vi "Read Write Script 2.vi"(5 "# of Words":i32, 6 "chip select (0)":u32, 7 "Write register":u8, 8 "error in (no error)":errorcluster, 9 "Write Data":u8[][](array[numeric]), 10 "delay in milliseconds (0)":u8, 11 "spi script reference in":T1) -> (0 "error out":errorcluster, 1 "script read index":u32, 3 "spi script reference out":T1)   [LabVIEW 2013]
uses:
  <vilib>/ni845x/ni845x.llb/ni845xSpiScriptControl.ctl
  <vilib>/ni845x/ni845x.llb/NI-845x SPI Script Ms Delay.vi
panel:
  out "data set":u8[](array[numeric])
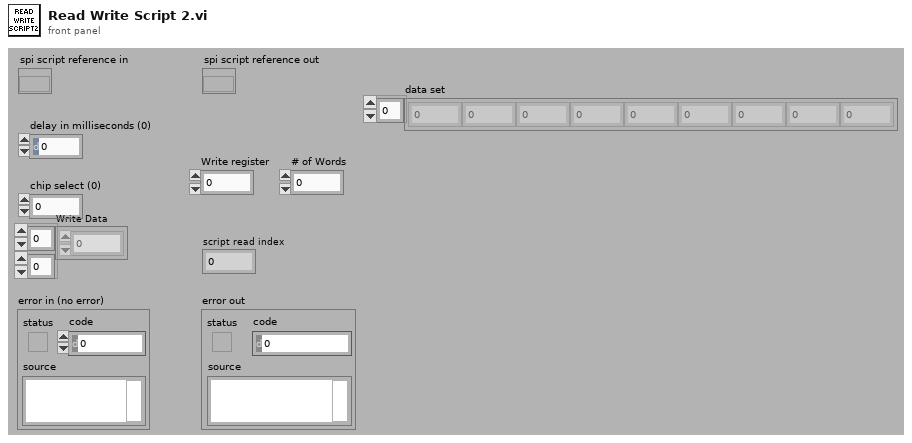
[diagram p1: front panel]
types:
  T1 = typedef "ni845xSpiScriptControl.ctl" = refnum<k20>
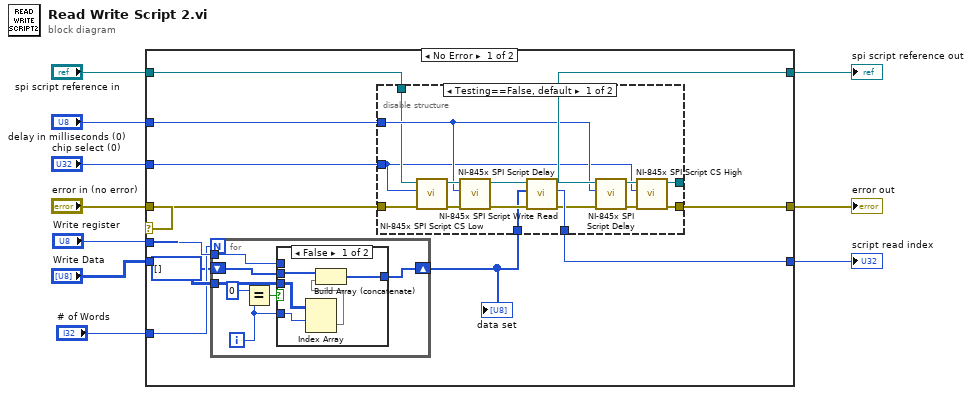
[diagram p0: block diagram]
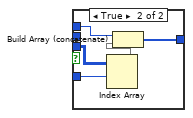
[diagram p2: hidden frame]
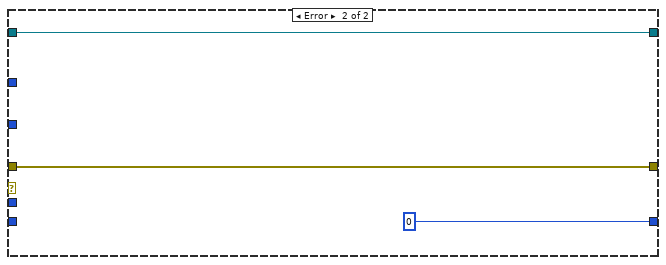
[diagram p4: hidden frame]
diagram:
  n1 = case shown="No Error" "error in (no error)" {
    tunnel: [w22 u32 0 ("script read index")] -> w10
    tunnel: [w21 w58] -> w9
    tunnel: [w20 w60] -> w8
    tunnel: "Write Data" -> [w14 _]
    tunnel: "delay in milliseconds (0)" -> [w19 _]
    tunnel: "error in (no error)" -> [w18 w60]
    tunnel: "spi script reference in" -> [w17 w58]
    tunnel: "chip select (0)" -> [w16 _]
    tunnel: "Write register" -> [w15 _]
    tunnel: "# of Words" -> [w12 _]
    frame No Error {
      n2 = for {
        N: w12 -> [_]
        tunnel: w15 -> [w29]
        tunnel: w14 -> [w26]
        shift-right: [w24] -> w13
        shift-left: u8[] [] -> [w23]
        i -> [w25]
        n3 = Equal?(x=u8 0, y=w25) -> (x = y?=w27:bool)
        n4 = case shown="False" w27 {
          tunnel: w29 -> [_ w39]
          tunnel: w26 -> [w33 w38]
          tunnel: w25 -> [w34 w37]
          tunnel: [w32 w35] -> w24
          tunnel: w23 -> [w31 _]
          frame False {
            n5 = Index Array(array=w33, index (row)=w34) -> (element=w30:u8[])  [unwired: 1 in]
            n6 = Build Array (concatenate)(w31, w30) -> (w32:u8[])
          }
          frame True {
            n7 = Index Array(array=w38, index (row)=w37) -> (element=w36:u8[])  [unwired: 1 in]
            n8 = Build Array (concatenate)(w39, w36) -> (w35:u8[])
          }
        }
      }
      "data set" <- w13
      n9 = disable-structure shown="Testing==False, default" {
        disable-tunnel: [w55 _] -> w22
        disable-tunnel: [w46 w56] -> w21
        disable-tunnel: [w45 w57] -> w20
        disable-tunnel: w13 -> [w44 _]
        disable-tunnel: w19 -> [w43 _]
        disable-tunnel: w18 -> [w42 w57]
        disable-tunnel: w17 -> [w41 w56]
        disable-tunnel: w16 -> [w40 _]
        frame condition #0 (active) {
          n10 = call <vilib>:"NI-845x SPI Script CS Low.vi"("error in (no error)"=w42, "chip select (0)"=w40, "spi script reference in"=w41) -> ("error out"=w49:errorcluster, "spi script reference out"=w50:T1)  [unwired: 7 in]
          n11 = call-poly <vilib>:"NI-845x SPI Script Delay.vi"("error in (no error)"=w49, "delay in milliseconds (0)"=w43, "spi script reference in"=w50) -> ("error out"=w47:errorcluster, "spi script reference out"=w48:T1)  [unwired: 7 in]
          n12 = call <vilib>:"NI-845x SPI Script Write Read.vi"("error in (no error)"=w47, "write data"=w44, "spi script reference in"=w48) -> ("error out"=w54:errorcluster, "script read index"=w55:u32, "spi script reference out"=w53:T1)  [unwired: 6 in]
          n13 = call-poly <vilib>:"NI-845x SPI Script Delay.vi"("error in (no error)"=w54, "delay in milliseconds (0)"=w43, "spi script reference in"=w53) -> ("error out"=w51:errorcluster, "spi script reference out"=w52:T1)  [unwired: 7 in]
          n14 = call <vilib>:"NI-845x SPI Script CS High.vi"("error in (no error)"=w51, "chip select (0)"=w40, "spi script reference in"=w52) -> ("error out"=w45:errorcluster, "spi script reference out"=w46:T1)  [unwired: 7 in]
        }
        frame condition #1 {
        }
      }
    }
    frame Error {
    }
  }
  "script read index" <- w10
  "spi script reference out" <- w9
  "error out" <- w8
